vi "Start experiment.vi"(7 "API Key":string, 8 "error in":errorcluster, 11 "Name of LAG SIM user":string) -> (0 "error out":errorcluster, 2 "Thread ID":i32, 3 "Experiment ID":i32)   [LabVIEW 2018]
uses:
  <vilib>/httpClient/POSTBuffer.vi
  <vilib>/httpClient/LabVIEWHTTPClient.lvlib
panel:
  out "Server response debug panel":string
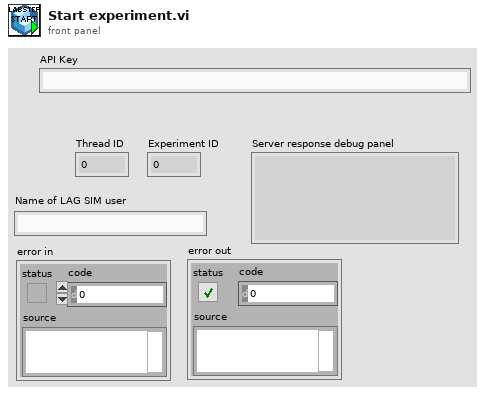
[diagram p1: front panel]
types:
  T1 = typedef "LabVIEWHTTPClient.lvlib/ClientHandle.ctl" = refnum<k1>
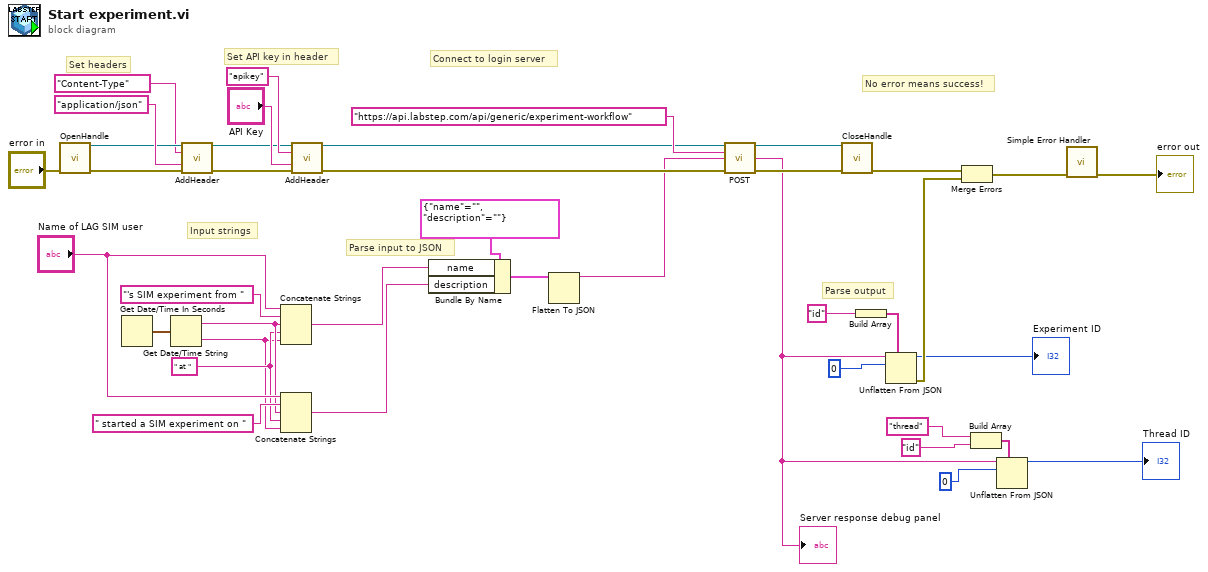
[diagram p0: block diagram]
diagram:
  w19 = " at " ("string")
  # "No error means success!"
  # "Parse output"
  # "Set API key in header"
  # "Input strings"
  # "Set headers"
  # "Connect to login server"
  # "Parse input to JSON"
  n1 = call <vilib>:"OpenHandle.vi"("error in (no error)"="error in") -> ("client handle out"=w38:T1, "error out"=w37:errorcluster)  [unwired: 13 in]
  n2 = Get Date/Time In Seconds() -> (seconds since 1Jan1904=w23:timestamp)
  n3 = Get Date/Time String(seconds (now)=w23) -> (date string=w20:string, time string=w18:string)  [unwired: 2 in]
  n4 = call <vilib>:"AddHeader.vi"("client handle"=w38, "header"="Content-Type", "value"="application/json", "error in (no error)"=w37) -> ("client handle out"=w27:T1, "error out"=w30:errorcluster)  [unwired: 10 in]
  n5 = Concatenate Strings("Name of LAG SIM user", "'s SIM experiment from " ("string"), w20, w19, w18) -> (w25:string)
  n6 = Concatenate Strings("Name of LAG SIM user", " started a SIM experiment on " ("string"), w20, w19, w18) -> (w17:string)
  n7 = call <vilib>:"AddHeader.vi"("client handle"=w27, "header"="apikey", "value"="API Key", "error in (no error)"=w30) -> ("client handle out"=w28:T1, "error out"=w29:errorcluster)  [unwired: 10 in]
  n8 = Bundle By Name(cluster=cluster{"name":string, "description":string} {"name"="", "description"=""}, "name"=w25, "description"=w17) -> (w36:cluster{"name":string, "description":string})
  n9 = Flatten To JSON(anything=w36) -> (JSON string=w26:string)  [unwired: 2 in, 1 out]
  n10 = call-poly <vilib>:"POST.vi"("client handle"=w28, "url"="https://api.labstep.com/api/generic/experiment-workflow", "buffer"=w26, "error in (no error)"=w29) -> ("client handle out"=w13:T1, "body"=w6:string, "error out"=w12:errorcluster)  [unwired: 8 in, 1 out]
  "Server response debug panel" <- w6
  n11 = call <vilib>:"CloseHandle.vi"("client handle"=w13, "error in (no error)"=w12) -> ("error out"=w10:errorcluster)  [unwired: 13 in]
  n12 = Build Array("id") -> (w15:string[])
  n13 = Unflatten From JSON(path=w15, JSON string=w6, type and defaults=0) -> (value=→"Experiment ID":i32, error out=w9:errorcluster)  [unwired: 4 in]
  n14 = Merge Errors(w10, w9) -> (w14:errorcluster)
  n15 = Build Array("thread" ("element"), "id") -> (w5:string[])
  n16 = Unflatten From JSON(path=w5, JSON string=w6, type and defaults=0) -> (value=→"Thread ID":i32)  [unwired: 4 in, 1 out]
  n17 = call <vilib>:"Simple Error Handler.vi"("error in (no error)"=w14) -> ("error out"=→"error out":errorcluster)  [unwired: 4 in, 4 out]
